vi "init.vi"(0 "Digital Input Test in":refnum<class "Digital Input Test.lvclass">, 1 "Value to Expect":T1, 2 "ConfigureILCStrategy":refnum<class "IConfigureILCStrategy.lvclass">, 3 "ReadILCStrategy":refnum<class "IReadILCStrategy.lvclass">, 4 "ILC":refnum<class "ILC.lvclass">, 5 "error in (no error)":errorcluster, 6 "Test Scenario":T2, 7 "Log":refnum<class "ITestLog.lvclass">, 8 "Signal Name":string) -> (14 "Digital Input Test out":refnum<class "Digital Input Test.lvclass">, 19 "error out":errorcluster)   [LabVIEW 2015, in "Digital Input Test.lvclass"]
uses:
  Digital Input Test.lvclass
  Model/TestLog/ITestLog/ITestLog.lvclass
  Typedefs/TestScenarioTypes.ctl
  Model/ConfigureILCStrategy/IConfigureILCStrategy/IConfigureILCStrategy.lvclass
  <userlib>/Common/ILC/ILC/ILC.lvclass
  Typedefs/Digital Signal Level.ctl
  Model/ReadILCStrategy/IReadILCStrategy/IReadILCStrategy.lvclass
  Digital Input Test.lvclass/Digital Input Test.ctl
  Typedefs/ILCBTTypedefs.lvlib
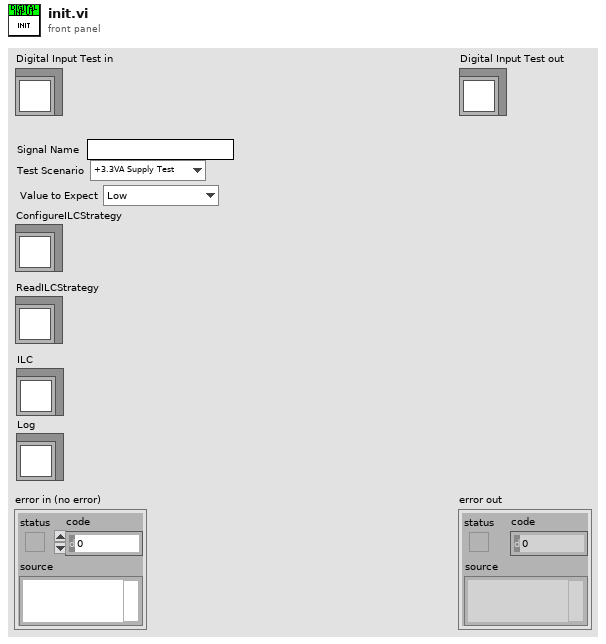
[diagram p1: front panel]
types:
  T1 = typedef "ILCBTTypedefs.lvlib/Digital Signal Level.ctl" = enum16{"Low", "High"}
  T2 = typedef "ILCBTTypedefs.lvlib/TestScenarioTypes.ctl" = enum16{"+3.3VA Supply Test", "+3.3VD Supply Test", "+5VA Supply Test", "+5VD Supply Test", "Unique ID Test", "TEDS Status Test", "LIMSW1_TTL Low Test", "LIMSW1_TTL High Test", "LIMSW2_TTL Low Test", "LIMSW2_TTL High Test", "Tachometer Test", "SSR_TTL Low Test", "SSR_TTL High Test", "SM_CW Low Test", "SM_CW High Test", "SM_CCW Low Test", "SM_CCW High Test", "SM_GPI Low Test", "SM_GPI High Test", "CW Motion Without Limit Test", "CW Motion With Limit Test", "CW Motion With Limit Interruption Test", "CW Motion on CCW Limit Test", "CCW Motion Without Limit Test", "CCW Motion With Limit Test", "CCW Motion With Limit Interruption Test", "CCW Motion on CW Limit Test", "RS232-TXD Low Test", "RS232-TXD High Test", "RS232-RTS Low Test", "RS232-RTS High Test", "RS232-RXD Low Test", "RS232-RXD High Test", "RS232-CTS Low Test", "RS232-CTS High Test", "Out_SS Low Test", "Out_SS High Test", "Out_SDI Low Test", "Out_SDI High Test", "Out_SCLK Low Test", "Out_SCLK High Test", "Reset Low Test", "Reset High Test", "1 Channel ADC Test", "3 Channel ADC Test", "5 Channel ADC Test", "Vref Test", "ROT Test", "DAC1 Test", "DAC2 Test", "DAC3 Test", "DAC4 Test", "BIAS Test", "EXC1 Test", "EXC2 Test", "EXC3 Test", "EXC4 Test"}
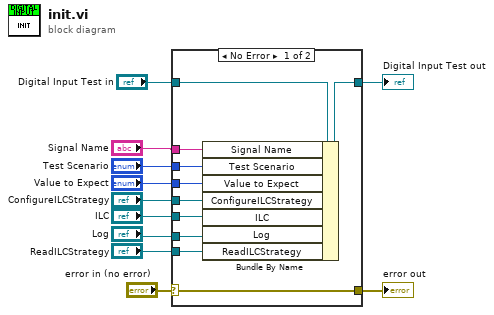
[diagram p0: block diagram]
diagram:
  n1 = case shown="No Error" "error in (no error)" {
    selector: "error in (no error)" -> [w21 w23]
    tunnel: [w21 w23] -> w10
    tunnel: [w15 w22] -> w8
    tunnel: "Digital Input Test in" -> [w20 w22]
    tunnel: "Signal Name" -> [w14 _]
    tunnel: "Test Scenario" -> [w13 _]
    tunnel: "ConfigureILCStrategy" -> [w17 _]
    tunnel: "ILC" -> [w18 _]
    tunnel: "Log" -> [w19 _]
    tunnel: "Value to Expect" -> [w16 _]
    tunnel: "ReadILCStrategy" -> [w12 _]
    frame No Error {
      n2 = Bundle By Name(cluster=w20, "Signal Name"=w14, "Test Scenario"=w13, "Value to Expect"=w16, "ConfigureILCStrategy"=w17, "ILC"=w18, "Log"=w19, "ReadILCStrategy"=w12) -> (w15:refnum<class "Digital Input Test.lvclass">)
    }
    frame Error {
    }
  }
  "error out" <- w10
  "Digital Input Test out" <- w8
